vi "oax_Load Shaft Centerline Data.vi"() -> (0 "error out":errorcluster, 1 "end position":i32, 2 "current position":i32, 3 "refnum":refnum<file>, 4 "channel info":T1[](array[typedef]) {"pregain" format="%.2f"; "weighting filter" items=["Linear", "A-weighting", "B-weighting", "C-weighting", "ITU-R 468-4", "Dolby", "CCITT", "C-message", "Wb", "Wc", "Wd", "We", "Wf", "Wh", "Wj", "Wk", "Wm", "AES17 20 kHz lowpass", "AES17 40 kHz lowpass", "AES17 20 kHz highpass", "AES17 40 kHz highpass"]; "dB reference" format="%^.1e"; "engineering units" items=["custom..."=0, "V"=1, "A"=21, "C"=30, "pC"=31, "s"=32, "-"=29, "Pa"=2, "N"=20, "g"=3, "m/s^2"=4, "m/s"=5, "m"=6, "mm/s"=12, "mm"=13, "micron/s"=14, "micron"=15, "in/s^2"=7, "in/s"=8, "in"=9, "mil/s"=10, "mil"=11, "rad/s^2"=16, "rad/s"=17, "rad"=18, "deg/s^2"=26, "deg/s"=27, "deg"=28, "RPM"=22, "cycle/s^2"=23, "Hz"=24, "cycle"=25, "strain"=19]; "sensor sensitivity" format="%#_5f"}, 5 "channel name":string[](array[string]), 6 "pulse / rev":i32)   [LabVIEW 2017]
doc: "Loads predefined shaft centerline data in a .ddt file."
uses:
  <vilib>/addons/_NISVFA/_Shared subVIs/Controls/svc_Channel Info.ctl
  <vilib>/addons/_NISVFA/_Shared subVIs/Controls/svc_Engineering Units Text Ring.ctl
  <vilib>/addons/_NISVFA/_Shared subVIs/Controls/svc_Weighting Filter Text Ring.ctl
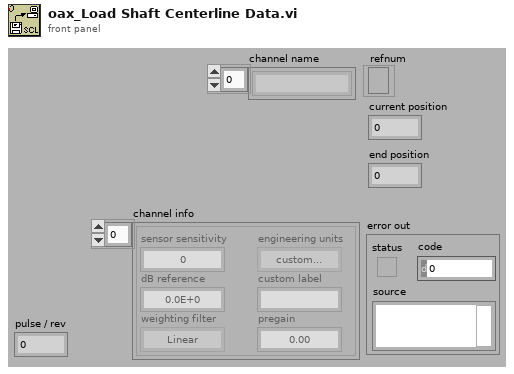
[diagram p1: front panel]
types:
  T1 = typedef "svc_Channel Info.ctl" = cluster{"sensor sensitivity":dbl, "engineering units":T2, "dB reference":dbl, "custom label":string, "weighting filter":T3, "pregain":dbl}
  T2 = typedef "svc_Engineering Units Text Ring.ctl" = u16
  T3 = typedef "svc_Weighting Filter Text Ring.ctl" = u16
  T4 = enum16{"open", "open or create", "create or replace", "create", "open (read only)"}
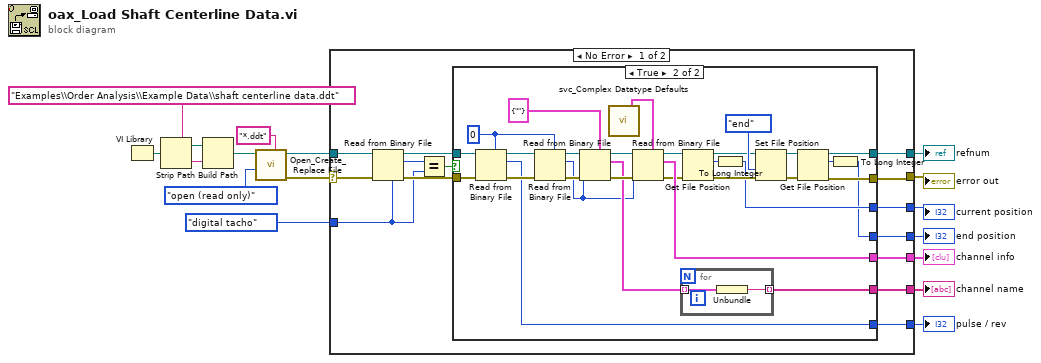
[diagram p0: block diagram]
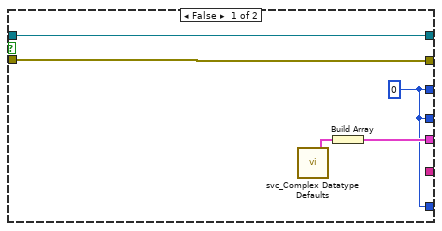
[diagram p2: hidden frame]
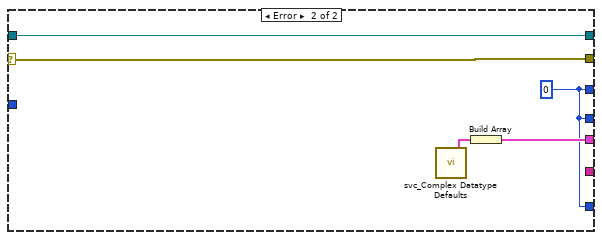
[diagram p3: hidden frame]
diagram:
  n1 = VI Library() -> (path=w14:path)
  n2 = Strip Path(path=w14) -> (stripped path=w13:path)  [unwired: 1 out]
  n3 = Build Path(base path=w13, name or relative path="Examples\\Order Analysis\\Example Data\\shaft centerline data.ddt") -> (appended path=w11:path)
  n4 = call <vilib>:"Open_Create_Replace File.vi"("pattern"="*.ddt", "function (open:0)"=T4."open (read only)", "file path"=w11) -> ("error out"=w9:errorcluster, "refnum"=w10:refnum<file>)  [unwired: 5 in, 2 out]
  n5 = case shown="No Error" w9 {
    selector: w9 -> [w27 w71]
    tunnel: [w21 w71] -> w7
    tunnel: w10 -> [w30 w70]
    tunnel: [w22 w70] -> w8
    tunnel: [w24 w68] -> w4
    tunnel: [w23 _] -> w3
    tunnel: [w20 w67] -> w6
    tunnel: [w19 w67] -> w5
    tunnel: enum16{"analog tacho", "digital tacho"}."digital tacho" -> [w18 _]
    tunnel: [w17 w67] -> w1
    frame No Error {
      n6 = Read from Binary File(5:w18, 8:w27, 11:w30) -> (0:w25:errorcluster, 2:w29:enum16{"analog tacho", "digital tacho"}, 3:w26:refnum<file>)  [unwired: 3 in, 1 out]
      n7 = Equal?(x=w29, y=w18) -> (x = y?=w28:bool)
      n8 = case shown="True" w28 {
        tunnel: w26 -> [w35 w63]
        tunnel: w25 -> [w34 w64]
        tunnel: [w32 w53] -> w24
        tunnel: [_ w56] -> w23
        tunnel: [w35 w46] -> w22
        tunnel: [w34 w45] -> w21
        tunnel: [w31 w44] -> w20
        tunnel: [w31 w43] -> w19
        tunnel: [w31 w36] -> w17
        frame False {
          w31 = 0 ("offset")
          n9 = call <vilib>:"svc_Complex Datatype Defaults.vi"() -> ("channel info"=w33:T1)  [unwired: 11 in, 8 out]
          n10 = Build Array(w33) -> (w32:T1[])
        }
        frame True {
          w52 = 0
          n11 = Read from Binary File(5:w52, 8:w64, 11:w63) -> (0:w60:errorcluster, 2:w36:i32, 3:w58:refnum<file>)  [unwired: 3 in, 1 out]
          n12 = Read from Binary File(5:w52, 8:w60, 11:w58) -> (0:w59:errorcluster, 2:w50:i32, 3:w57:refnum<file>)  [unwired: 3 in, 1 out]
          n13 = Read from Binary File(5:cluster{"ch0 string":string} {"ch0 string"=""}, 8:w59, 10:w50, 11:w57) -> (0:w62:errorcluster, 2:w54:cluster{"ch0 string":string}[], 3:w61:refnum<file>)  [unwired: 2 in, 1 out]
          n14 = call <vilib>:"svc_Complex Datatype Defaults.vi"() -> ("channel info"=w47:T1)  [unwired: 11 in, 8 out]
          n15 = Read from Binary File(5:w47, 8:w62, 10:w50, 11:w61) -> (0:w38:errorcluster, 2:w53:T1[], 3:w39:refnum<file>)  [unwired: 2 in, 1 out]
          n16 = for {
            tunnel: w54 -> [w66] mode=indexing
            tunnel: [w65] -> w56 mode=indexing
            n17 = Unbundle(w66) -> ("ch0 string"=w65:string)
          }
          n18 = Get File Position(4:w38, 7:w39) -> (0:w49:errorcluster, 2:w37:i64, 3:w48:refnum<file>)
          n19 = To Long Integer(number=w37) -> (32bit integer=w44:i32)
          n20 = Set File Position(refnum=w48, from (0:start)=enum16{"start", "end", "current"}."end" ("pos mode (0:2)"), error in=w49) -> (refnum out=w42:refnum<file>, error out=w41:errorcluster)  [unwired: 1 in]
          n21 = Get File Position(4:w41, 7:w42) -> (0:w45:errorcluster, 2:w40:i64, 3:w46:refnum<file>)
          n22 = To Long Integer(number=w40) -> (32bit integer=w43:i32)
        }
      }
    }
    frame Error {
      w67 = 0 ("offset")
      n23 = call <vilib>:"svc_Complex Datatype Defaults.vi"() -> ("channel info"=w69:T1)  [unwired: 11 in, 8 out]
      n24 = Build Array(w69) -> (w68:T1[])
    }
  }
  "refnum" <- w8
  "error out" <- w7
  "current position" <- w6
  "end position" <- w5
  "channel info" <- w4
  "channel name" <- w3
  "pulse / rev" <- w1
